vi "Rotated Rectangle.vi"(8 "Angle":dbl, 10 "Rectangle":cluster{i32, i32, i32, i32}) -> (2 "x*y":cluster{dbl, dbl}[](array[cluster]))   [LabVIEW 2019]
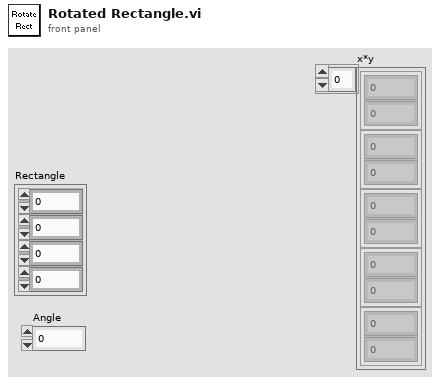
[diagram p1: front panel]
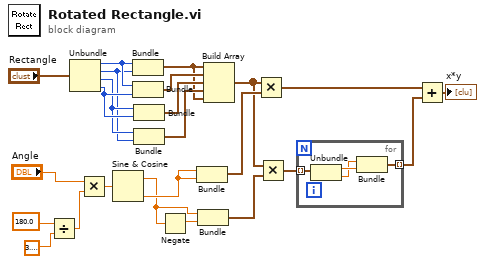
[diagram p0: block diagram]
diagram:
  n1 = Divide(x=180.0, y=3.141592653589793) -> (x/y=w12:dbl)
  n2 = Unbundle("Rectangle") -> (w18:i32, w16:i32, w17:i32, w23:i32)
  n3 = Multiply(x="Angle", y=w12) -> (x*y=w10:dbl)
  n4 = Sine & Cosine(0:w10) -> (1:w3:dbl, 2:w5:dbl)
  n5 = Bundle(w18, w16) -> (w19:cluster{i32, i32})  [unwired: 1 in]
  n6 = Bundle(w18, w23) -> (w22:cluster{i32, i32})  [unwired: 1 in]
  n7 = Bundle(w17, w23) -> (w21:cluster{i32, i32})  [unwired: 1 in]
  n8 = Bundle(w17, w16) -> (w20:cluster{i32, i32})  [unwired: 1 in]
  n9 = Negate(x=w3) -> (-x=w4:dbl)
  n10 = Bundle(w5, w5) -> (w15:cluster{dbl, dbl})  [unwired: 1 in]
  n11 = Bundle(w3, w4) -> (w8:cluster{dbl, dbl})  [unwired: 1 in]
  n12 = Build Array(w19, w22, w21, w20, w19) -> (w9:cluster{i32, i32}[])
  n13 = Multiply(x=w9, y=w15) -> (x*y=w7:cluster{dbl, dbl}[])
  n14 = Multiply(x=w9, y=w8) -> (x*y=w2:cluster{dbl, dbl}[])
  n15 = for {
    tunnel: w2 -> [w28] mode=indexing
    tunnel: [w25] -> w1 mode=indexing
    n16 = Unbundle(w28) -> (w27:dbl, w26:dbl)
    n17 = Bundle(w26, w27) -> (w25:cluster{dbl, dbl})  [unwired: 1 in]
  }
  n18 = Add(x=w7, y=w1) -> (x+y=→"x*y":cluster{dbl, dbl}[])
